vi "Test Copy Image to Pixmap No Mask ARGB.vi"(8 "error in (no error)":errorcluster, 11 "Test Case In":refnum<class "01_Image.lvclass">) -> (0 "error out":errorcluster, 3 "Test Case Out":refnum<class "01_Image.lvclass">)   [LabVIEW 2020, in "test.lvlib" / "01_Image.lvclass"]
uses:
  01_Image.lvclass
  C:/Program Files (x86)/National Instruments/LabVIEW 2026/vi.lib/Astemes/LUnit/Test Case.lvclass
  common/Image Size (Integer).ctl
  <vilib>/Astemes/LUnit/Test Case.lvclass/Test Case.ctl
  image/Copy Image to Pixmap (ARGB).vi
  4993e8ee-a06a-463a-9684-69129f64d5ce.vi
  image/New Image.vi
  image/New Image (ARGB Preallocated).vi
  image/Copy Array to Image.vi
  image/Copy Array to Image (ARGB).vi
  image/Copy Image to Pixmap (ARGB).vi/5c639587-cf36-4d54-93d9-e654c7c24c6e.vi
  <vilib>/Astemes/LUnit/Core/LUnit Test Case/Private/Append Pass Result.vi
  <vilib>/Astemes/LUnit/Core/LUnit Test Case/Private/Append Fail Result.vi
  4993e8ee-a06a-463a-9684-69129f64d5ce.vi/9c5d11cd-9439-4240-a1ee-d9baace9c924.vi
  image/New Image (ARGB Preallocated).vi/3321fa97-f432-4e1e-8db9-a0df79aed21b.vi
  image/ARGB Colour to U32 Pixel Value.vi
  <vilib>/Astemes/LUnit/Core/LUnit Test Case/Private/Run In UI.vi
  <vilib>/Utility/error.llb/Clear Errors.vi
  <vilib>/Utility/error.llb/Error Cluster From Error Code.vi
  <vilib>/picture/pixmap.llb/Flatten Pixmap.vi
  common/common.lvlib
  image/image.lvlib
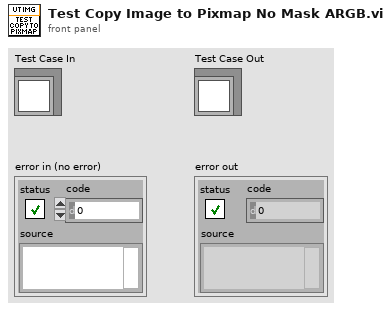
[diagram p1: front panel]
types:
  T1 = typedef "common.lvlib/Image Size (Integer).ctl" = cluster{"Width":u16, "Height":u16}
  T2 = typedef "image.lvlib/ARGB Image.ctl" = refnum<data-value>
  T3 = typedef "imagedata.ctl" = cluster{"image type":i32, "image depth":i32, "image":u8[], "mask":u8[], "colors":u32[], "Rectangle":cluster{"left":i16, "top":i16, "right":i16, "bottom":i16}}
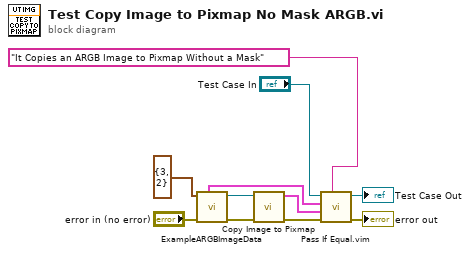
[diagram p0: block diagram]
diagram:
  n1 = call "ExampleARGBImageData.vi"("error in (no error)"="error in (no error)", "Image Size"=T1 {"Width"=3, "Height"=2} ("Preallocated Image Size (Default - 0,0)")) -> ("error out"=w7:errorcluster, "Data Value Reference out"=w4:T2, "ARGB Pixmap Data"=w2:T3)  [unwired: 6 in, 1 out]
  n2 = call-poly "Copy Image to Pixmap.vi"("error in (no error)"=w7, "ARGB Image Source in"=w4) -> ("error out"=w3:errorcluster, "Pixmap Image Data"=w1:T3)  [unwired: 8 in]
  n3 = call "Pass If Equal.vim"("Description"="It Copies an ARGB Image to Pixmap Without a Mask", "error in (no error)"=w3, "Actual"=w1, "Expected"=w2, "LUnit Test Case In"="Test Case In") -> ("error out"=→"error out":errorcluster, "LUnit Test Case Out"=→"Test Case Out":refnum<class "01_Image.lvclass">)  [unwired: 5 in]
